vi "TicTacToev3.vi"() -> ()   [LabVIEW 2020]
panel:
  out "Human(GREEN) Win":dbl
  out "Computer(RED)Win":dbl
  in  "Numeric":i32
  out "Who's Tern ?":bool
  in  "LEVEL":i32(slide)=3000 scale=5.0..1.0
  in  "START GAME":bool
  in  "Boolean":bool
  in  "Boolean 3":bool
  in  "Boolean 4":bool
  in  "Boolean 5":bool
  in  "Boolean 6":bool
  in  "Boolean 7":bool
  in  "Boolean 8":bool
  in  "Boolean 9":bool
  in  "Boolean 2":bool
  in  "Turn 2":bool
  out "Turn":string
  out "Human Won":bool
  out "Computer Won":bool
  out "XO array":string[][](array[string])
  out "No one Won":bool
  out "Tie":bool
  in  "STOP GAME":bool
  out "Tank":i32(slide)
  out "Tank 2":i32(slide)
  out "players":dbl format="%#g"
  out "Game Over":bool
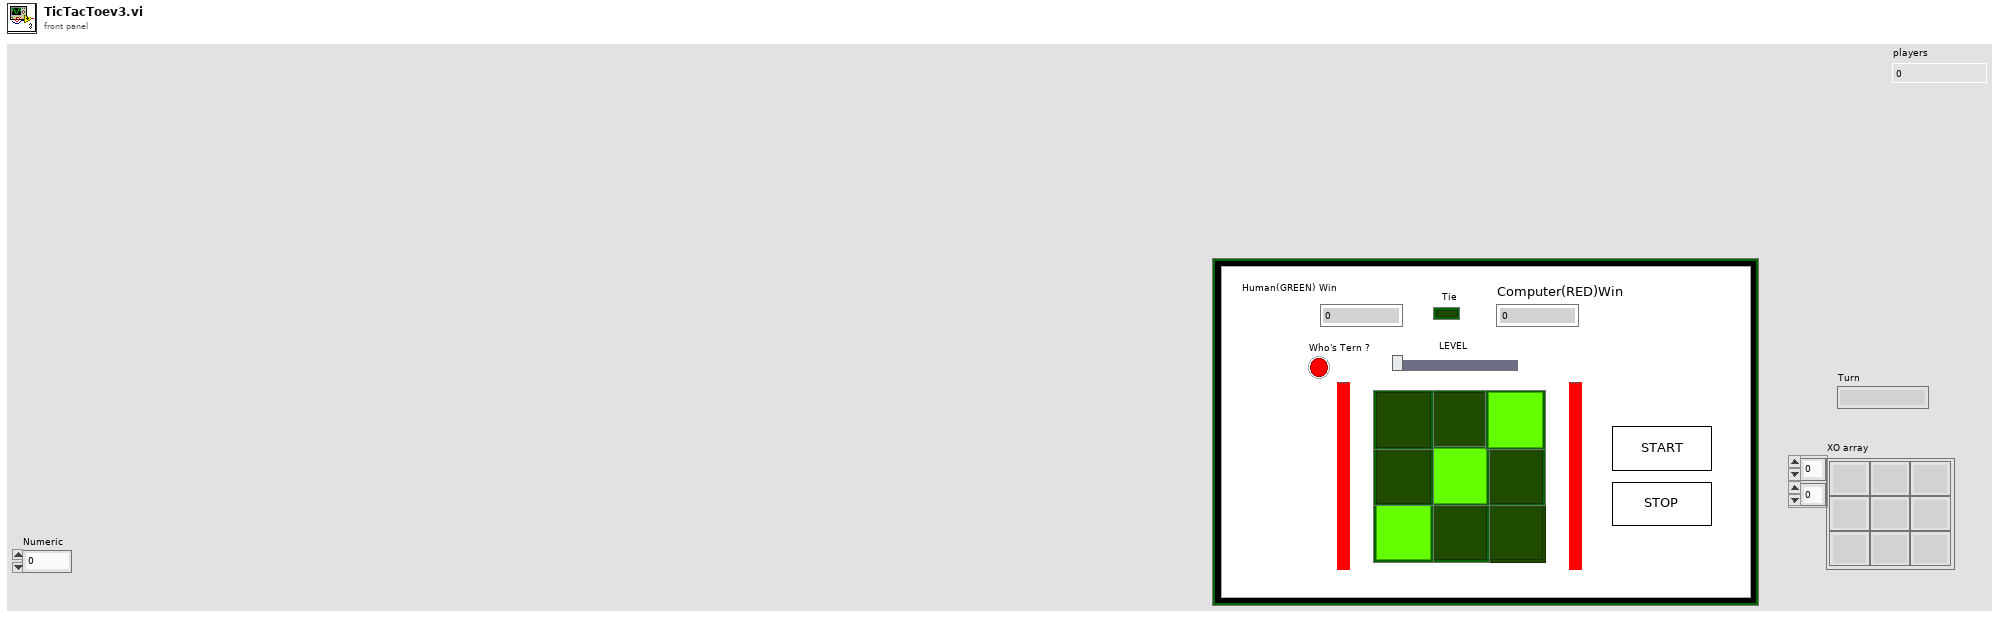
[diagram p1: front panel]
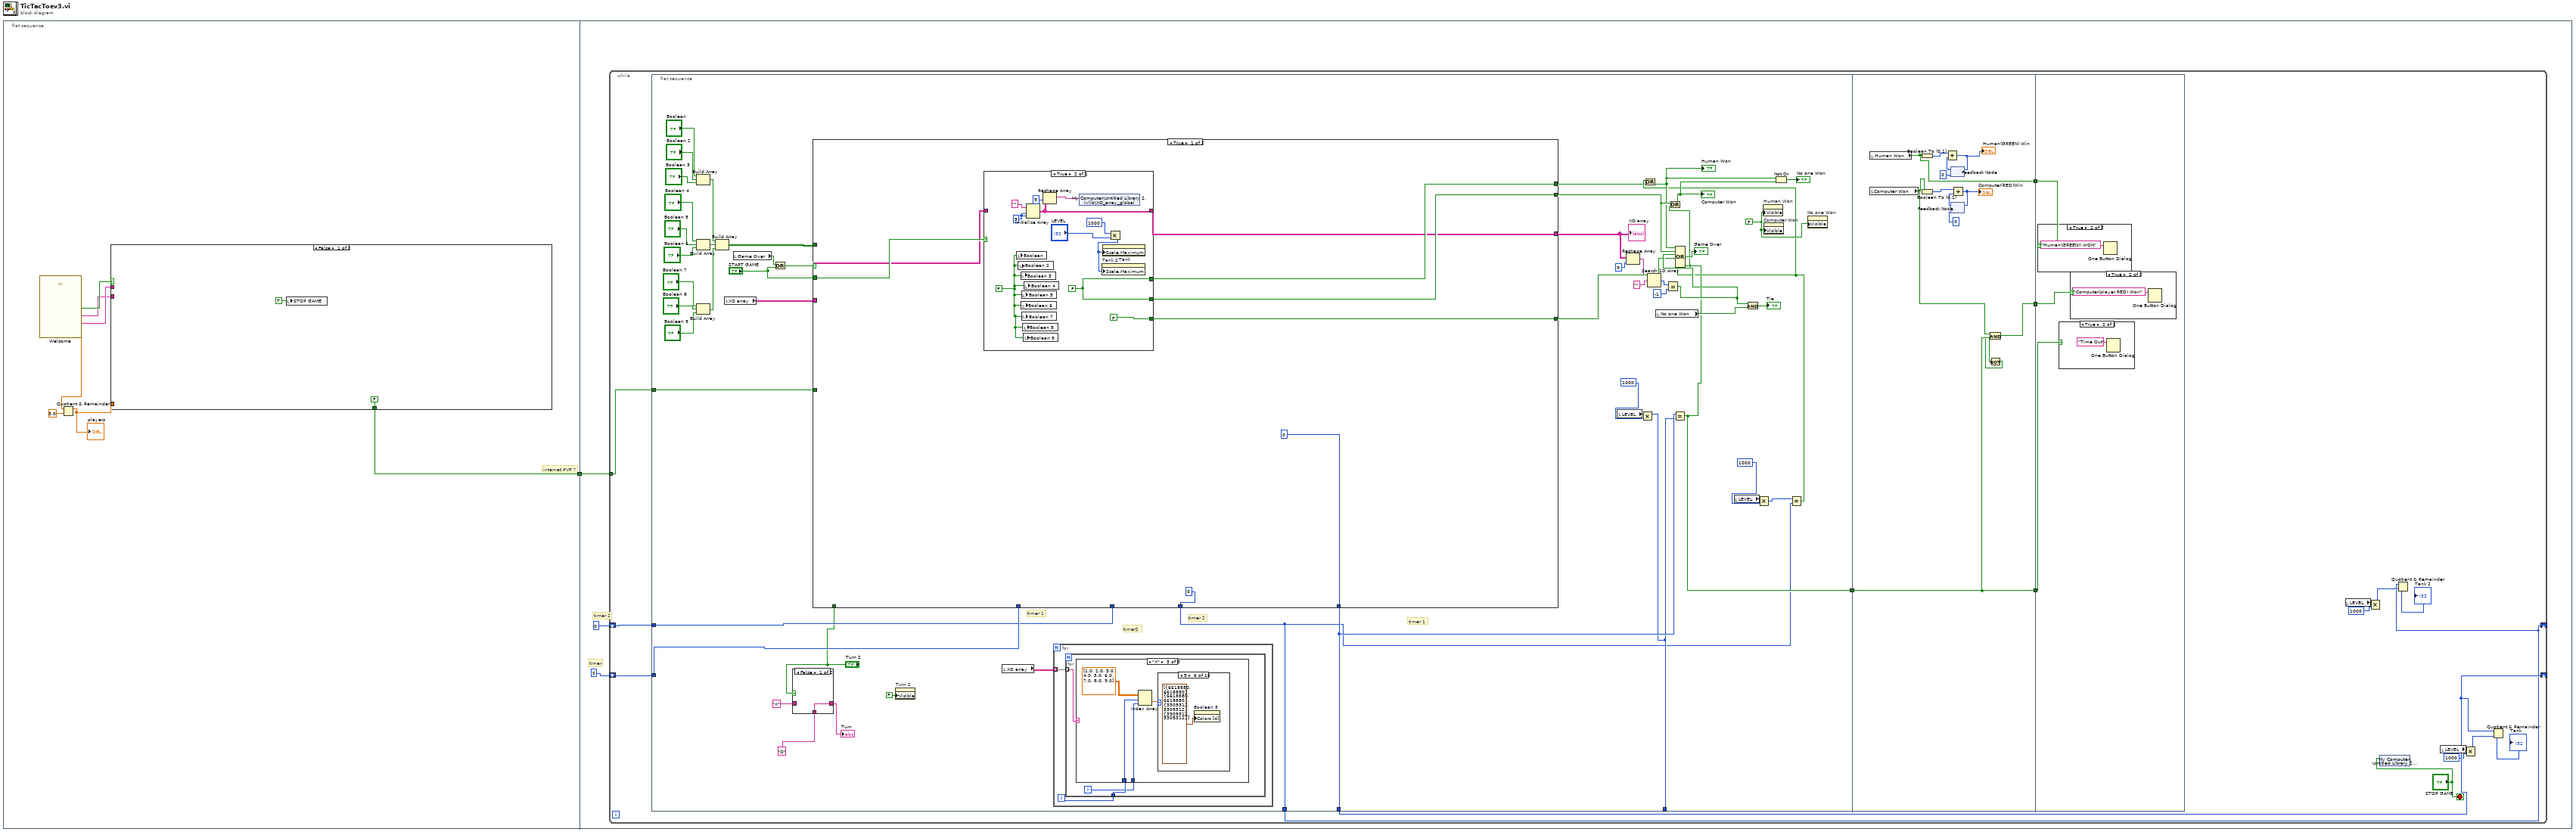
[diagram p0: block diagram]
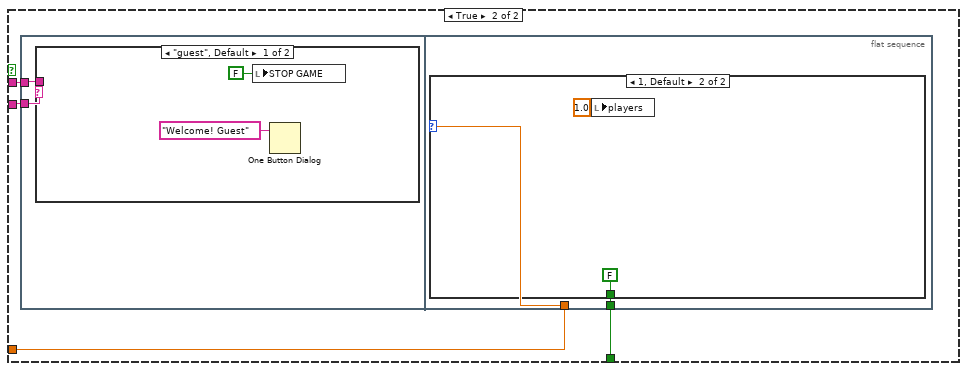
[diagram p2: hidden frame]
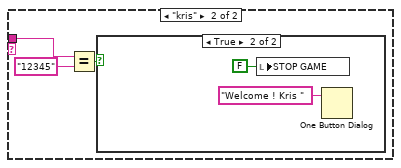
[diagram p3: hidden frame]
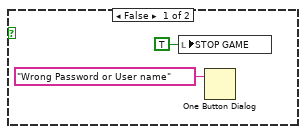
[diagram p4: hidden frame]
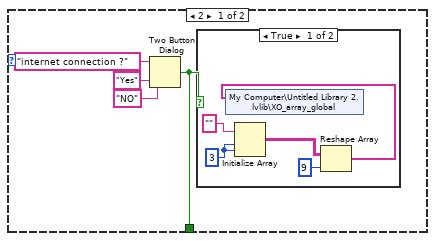
[diagram p5: hidden frame]
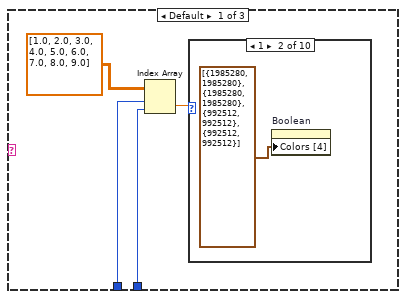
[diagram p7: hidden frame]
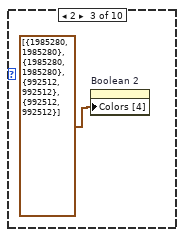
[diagram p9: hidden frame]
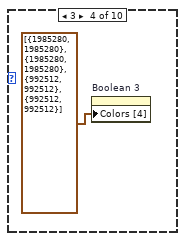
[diagram p10: hidden frame]
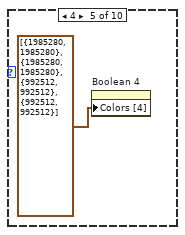
[diagram p11: hidden frame]
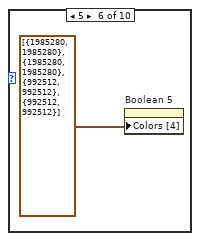
[diagram p12: hidden frame]
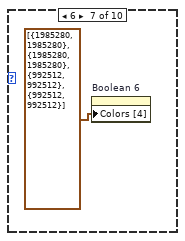
[diagram p13: hidden frame]
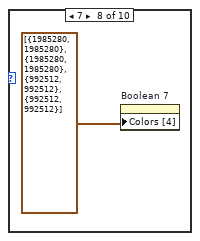
[diagram p14: hidden frame]
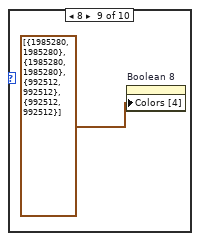
[diagram p15: hidden frame]
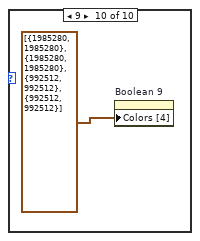
[diagram p16: hidden frame]
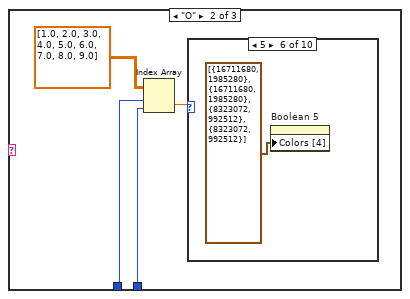
[diagram p17: hidden frame]
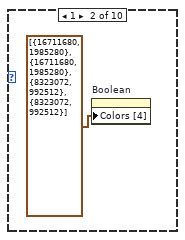
[diagram p19: hidden frame]
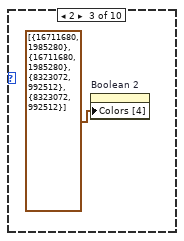
[diagram p20: hidden frame]
diagram:
  n1 = flat-sequence {
    tunnel: [w2] -> w1
    tunnel: w1 -> [w39]
    frame #0 {
      # "internet PVP ?"
      n2 = call "Welcome"() -> ("players(1 or 2 )"=w8:dbl, "password"=w5:string, "name"=w4:string, "OK"=w7:bool)  [unwired: 15 in, 1 out]
      n3 = Quotient & Remainder(x=w8, y=3.0) -> (x-y*floor(x/y)=w3:dbl)  [unwired: 1 out]
      "players" <- w3
      n4 = case shown="False" w7 {
        tunnel: w4 -> [_ w14]
        tunnel: w5 -> [_ w13]
        tunnel: w3 -> [_ w12]
        tunnel: [FALSE ("T button?") w11] -> w2
        frame False {
          n5 = local write "STOP GAME"(TRUE ("STOP GAME")) -> ()
        }
        frame True {
          n6 = flat-sequence {
            tunnel: w14 -> [w16]
            tunnel: w13 -> [w15]
            tunnel: w12 -> [w27]
            tunnel: [w26] -> w11
            frame #0 {
              n7 = case shown="\"guest\", Default" w16 {
                tunnel: w15 -> [_ w21]
                frame "guest", Default {
                  n8 = local write "STOP GAME"(FALSE ("STOP GAME")) -> ()
                  n9 = One Button Dialog(message="Welcome! Guest") -> ()  [unwired: 1 in, 1 out]
                }
                frame "kris" {
                  n10 = Equal?(x=w21, y="12345") -> (x = y?=w19:bool)
                  n11 = case shown="True" w19 {
                    frame False {
                      n12 = local write "STOP GAME"(TRUE ("STOP GAME")) -> ()
                      n13 = One Button Dialog(message="Wrong Password or User name") -> ()  [unwired: 1 in, 1 out]
                    }
                    frame True {
                      n14 = local write "STOP GAME"(FALSE ("STOP GAME")) -> ()
                      n15 = One Button Dialog(message="Welcome ! Kris ") -> ()  [unwired: 1 in, 1 out]
                    }
                  }
                }
              }
            }
            frame #1 {
              n16 = case shown="1, Default" w27 {
                tunnel: [w28 FALSE ("T button?")] -> w26
                frame 2 {
                  n17 = Two Button Dialog(message="internet connection ?", 1:"NO" ("F button name (\"Cancel\")"), 2:"Yes" ("T button name (\"OK\")")) -> (T button?=w28:bool)
                  n18 = case shown="True" w28 {
                    frame True {
                      w36 = 3
                      n19 = Initialize Array("", w36, w36) -> (w33:string[][])
                      n20 = Reshape Array(w33, 9 ("dimension size")) -> (w32:string[])
                      n21 = shared-variable "My Computer\\Untitled Library 2.lvlib\\XO_array_global"(w32) -> ()  [unwired: 1 in, 1 out]
                    }
                    frame False {
                    }
                  }
                }
                frame 1, Default {
                  n22 = local write "players"(1.0 ("players")) -> ()
                }
              }
            }
          }
        }
      }
    }
    frame #1 {
      # "timer 2"
      # "timer"
      n23 = while {
        shift-right: [w55] -> _
        shift-left: 0 -> [w57]
        shift-right: [w44] -> _
        shift-left: 0 -> [w49]
        tunnel: w39 -> [w42]
        stop <- "STOP GAME" stop-if-true
        n24 = flat-sequence {
          tunnel: [w75] -> w55
          tunnel: [w73] -> w53
          tunnel: [w71] -> _
          tunnel: w57 -> [w76]
          tunnel: w49 -> [w69]
          tunnel: [w65] -> w44
          tunnel: w42 -> [w61]
          tunnel: [w323] -> w59
          tunnel: [w326] -> w58
          tunnel: [w325] -> w54
          tunnel: w53 -> [w325]
          tunnel: w59 -> [w337]
          tunnel: w58 -> [w336]
          tunnel: w54 -> [w335]
          frame #0 {
            w78 = FALSE ("Visible")
            # "timer 1"
            # "timer 2"
            # "timer 1"
            # "timer2"
            n25 = Build Array("Boolean", "Boolean 2", "Boolean 3") -> (w110:bool[])
            n26 = Build Array("Boolean 4", "Boolean 5", "Boolean 6") -> (w111:bool[])
            n27 = Build Array("Boolean 7", "Boolean 8", "Boolean 9") -> (w112:bool[])
            n28 = Build Array(w110, w111, w112) -> (w102:bool[][])
            n29 = local read "XO array"() -> (w101:string[][])
            n30 = local read "Game Over"() -> (w94:bool)
            n31 = Or(x=w94, y="START GAME") -> (x .or. y?=w93:bool)
            n32 = case shown="False" "Turn 2" {
              tunnel: "X" -> [_ w158]
              tunnel: [w157 w158] -> w99
              tunnel: "O" ("x") -> [w157 _]
              frame False {
              }
              frame True {
              }
            }
            "Turn" <- w99
            n33 = case shown="True" w93 {
              tunnel: w102 -> [_ w202]
              tunnel: w101 -> [w165 w181]
              tunnel: "Turn 2" -> [_ w201]
              tunnel: "START GAME" -> [w166 _]
              tunnel: [w164 w194] -> w80
              tunnel: [w163 w193] -> w79
              tunnel: [w162 w192] -> w83
              tunnel: [w161 FALSE] -> w77
              tunnel: w76 -> [_ w190]
              tunnel: [0 w189] -> w75
              tunnel: w69 -> [_ w188]
              tunnel: [0 w187] -> w65
              tunnel: w61 -> [_ w183]
              frame True {
                n34 = case shown="True" w166 {
                  tunnel: [w169 w172] -> w162
                  tunnel: [w168 w179] -> w163
                  tunnel: [w168 w179] -> w164
                  tunnel: w165 -> [w169 _]
                  tunnel: [TRUE FALSE] -> w161
                  frame False {
                    w168 = FALSE
                  }
                  frame True {
                    w177 = FALSE
                    w179 = FALSE
                    w178 = 3
                    n35 = local write "Boolean"(w177) -> ()
                    n36 = local write "Boolean 2"(w177) -> ()
                    n37 = local write "Boolean 3"(w177) -> ()
                    n38 = local write "Boolean 6"(w177) -> ()
                    n39 = local write "Boolean 5"(w177) -> ()
                    n40 = local write "Boolean 7"(w177) -> ()
                    n41 = local write "Boolean 8"(w177) -> ()
                    n42 = local write "Boolean 9"(w177) -> ()
                    n43 = local write "Boolean 4"(w177) -> ()
                    n44 = Initialize Array("", w178, w178) -> (w172:string[][])
                    n45 = Reshape Array(w172, 9 ("dimension size")) -> (w171:string[])
                    n46 = shared-variable "My Computer\\Untitled Library 2.lvlib\\XO_array_global"(w171) -> ()  [unwired: 1 in, 1 out]
                    n47 = Multiply(x=1000, y="LEVEL") -> (x*y=w173:i32)
                    n48 = property on="Tank 2" class="Slide (strict)"("Scale.Maximum"=w173) -> ()  [unwired: 2 in, 2 out]
                    n49 = property on="Tank" class="Slide (strict)"("Scale.Maximum"=w173) -> ()  [unwired: 2 in, 2 out]
                  }
                }
              }
              frame False {
                n50 = local read "Turn"() -> (w182:string)
                n51 = shared-variable "My Computer\\Untitled Library 2.lvlib\\Turn_string"(w182) -> ()  [unwired: 1 in, 1 out]
                n52 = Equal?(x=w182, y="O") -> (x = y?=w185:bool)
                n53 = case shown="False" w185 {
                  frame False {
                    n54 = property on="Who's Tern ?" class="Bool (strict)"("Colors [4]"=cluster{u32, u32}[] [{6618880, 6618880}]) -> ()  [unwired: 2 in, 2 out]
                  }
                  frame True {
                    n55 = property on="Who's Tern ?" class="Bool (strict)"("Colors [4]"=cluster{u32, u32}[] [{16711680, 16711680}]) -> ()  [unwired: 2 in, 2 out]
                  }
                }
                n56 = case shown="False" w201 {
                  selector: w201 -> [w209 _]
                  tunnel: w202 -> [w216 w292]
                  tunnel: w181 -> [w218 w291]
                  tunnel: [w219 w284] -> w192
                  tunnel: w182 -> [w215 w290]
                  tunnel: w190 -> [w211 w288]
                  tunnel: [w214 w287] -> w189
                  tunnel: w188 -> [w213 _]
                  tunnel: [w212 0] -> w187
                  tunnel: w183 -> [w210 _]
                  frame False {
                    n57 = local read "players"() -> (w217:dbl)
                    n58 = case shown="2" w217 {
                      tunnel: [w225 w281] -> w219
                      tunnel: w218 -> [w228 w280]
                      tunnel: w216 -> [w226 _]
                      tunnel: w215 -> [w227 _]
                      tunnel: w213 -> [w224 _]
                      tunnel: [0 0] -> w214
                      tunnel: [w223 0] -> w212
                      tunnel: w211 -> [_ _]
                      tunnel: w210 -> [w221 _]
                      tunnel: w209 -> [w220 _]
                      frame 2 {
                        # "connect to timer2"
                        n59 = case shown="True" w221 {
                          tunnel: w228 -> [_ w245]
                          tunnel: w227 -> [_ w244]
                          tunnel: w226 -> [_ w243]
                          tunnel: [w231 w242] -> w225
                          tunnel: w224 -> [_ w241]
                          tunnel: ["Numeric" w240] -> w223
                          tunnel: w220 -> [w229 _]
                          frame True {
                            n60 = flat-sequence {
                              tunnel: w229 -> [w232]
                              tunnel: [w238] -> w231
                              frame #0 {
                                n61 = shared-variable "My Computer\\Untitled Library 2.lvlib\\Internet_PVP"(TRUE ("Internet_PVP")) -> ()  [unwired: 1 in, 1 out]
                                n62 = shared-variable "My Computer\\Untitled Library 2.lvlib\\Turn"(w232) -> ()  [unwired: 1 in, 1 out]
                                n63 = shared-variable "My Computer\\Untitled Library 2.lvlib\\timer_2"() -> (w233:i32)  [unwired: 1 in, 1 out]
                                n64 = local write "Numeric"(w233) -> ()
                              }
                              frame #1 {
                                n65 = shared-variable "My Computer\\Untitled Library 2.lvlib\\XO_array_global"() -> (w239:string[])  [unwired: 1 in, 1 out]
                                n66 = shared-variable "My Computer\\Untitled Library 2.lvlib\\Client_end"() -> (w235:bool)  [unwired: 1 in, 1 out]
                                n67 = local write "Turn 2"(w235) -> ()
                                n68 = Reshape Array(w239, 3 ("dimension size"), 3 ("dimension size")) -> (w238:string[][])
                              }
                            }
                          }
                          frame False {
                            w246 = 3
                            n69 = for {
                              N: w246 -> [_]
                              tunnel: w246 -> [w253]
                              tunnel: w243 -> [w252] mode=indexing
                              tunnel: w245 -> [w251] mode=indexing
                              tunnel: [w250] -> w242 mode=indexing
                              tunnel: w244 -> [w249]
                              tunnel: w241 -> [w248]
                              tunnel: [w247] -> w240
                              n70 = for {
                                N: w253 -> [_]
                                tunnel: w252 -> [w263] mode=indexing
                                tunnel: w251 -> [w260] mode=indexing
                                tunnel: w249 -> [w258]
                                tunnel: [w259] -> w250 mode=indexing
                                tunnel: w248 -> [w255]
                                tunnel: [w254] -> w247
                                n71 = Not Equal?(x=w260, y="X") -> (x != y?=w264:bool)
                                n72 = Not Equal?(x="O", y=w260) -> (x != y?=w265:bool)
                                n73 = And(x=w265, y=w264) -> (x .and. y?=w262:bool)
                                n74 = local read "Turn 2"() -> (w257:bool)
                                n75 = And(x=w263, y=w262) -> (x .and. y?=w261:bool)
                                n76 = case shown="True" w261 {
                                tunnel: w260 -> [w271 _]
                                tunnel: [w271 w273] -> w259
                                tunnel: w258 -> [_ w273]
                                tunnel: [w270 w274] -> w256
                                tunnel: w257 -> [w270 w275]
                                tunnel: w255 -> [w269 _]
                                tunnel: [w268 0] -> w254
                                frame False {
                                n77 = Increment(x=w269) -> (x+1=w268:i32)
                                }
                                frame True {
                                n78 = Not(x=w275) -> (.not. x?=w274:bool)
                                }
                                }
                                n79 = local write "Turn 2"(w256) -> ()
                              }
                            }
                          }
                        }
                      }
                      frame 1, Default {
                        n80 = local read "Turn 2"() -> (w279:bool)
                        n81 = call "AI algorithm(SubVI).vi"("Turn"=w279, "XO array"=w280) -> ("Turn 2"=w278:bool, "XO array 2"=w281:string[][])
                        n82 = local write "Turn 2"(w278) -> ()
                      }
                    }
                  }
                  frame True {
                    w289 = 3
                    n83 = for {
                      N: w289 -> [_]
                      tunnel: w289 -> [w299]
                      tunnel: w292 -> [w298] mode=indexing
                      tunnel: w291 -> [w297] mode=indexing
                      tunnel: [w296] -> w284 mode=indexing
                      tunnel: w290 -> [w295]
                      tunnel: w288 -> [w294]
                      tunnel: [w293] -> w287
                      n84 = for {
                        N: w299 -> [_]
                        tunnel: w298 -> [w309] mode=indexing
                        tunnel: w297 -> [w307] mode=indexing
                        tunnel: w295 -> [w305]
                        tunnel: [w306] -> w296 mode=indexing
                        tunnel: w294 -> [w301]
                        tunnel: [w300] -> w293
                        n85 = Not Equal?(x=w307, y="X") -> (x != y?=w310:bool)
                        n86 = Not Equal?(x="O", y=w307) -> (x != y?=w311:bool)
                        n87 = And(x=w311, y=w310) -> (x .and. y?=w308:bool)
                        n88 = local read "Turn 2"() -> (w303:bool)
                        n89 = And(x=w309, y=w308) -> (x .and. y?=w302:bool)
                        n90 = case shown="False" w302 {
                          tunnel: w307 -> [w317 _]
                          tunnel: [w317 w319] -> w306
                          tunnel: w305 -> [_ w319]
                          tunnel: [w316 w320] -> w304
                          tunnel: w303 -> [w316 w321]
                          tunnel: w301 -> [w315 _]
                          tunnel: [w314 0] -> w300
                          frame False {
                            n91 = Increment(x=w315) -> (x+1=w314:i32)
                          }
                          frame True {
                            n92 = Not(x=w321) -> (.not. x?=w320:bool)
                          }
                        }
                        n93 = local write "Turn 2"(w304) -> ()
                      }
                    }
                    n94 = shared-variable "My Computer\\Untitled Library 2.lvlib\\timer_2"(0 ("timer_2")) -> ()  [unwired: 1 in, 1 out]
                    n95 = Reshape Array(w284, 9 ("dimension size")) -> (w282:string[])
                    n96 = shared-variable "My Computer\\Untitled Library 2.lvlib\\XO_array_global"(w282) -> ()  [unwired: 1 in, 1 out]
                  }
                }
                n97 = call "CheckWinDiag(SubVI).vi"("Array"=w192) -> ("x .or. y?"=w199:bool)  [unwired: 10 in]
                n98 = Transpose 2D Array(2D array=w192) -> (transposed array=w200:string[][])
                n99 = call "CheckWinRow(SubVI).vi"("Array"=w192) -> ("x .or. y? 2"=w198:bool)  [unwired: 10 in]
                n100 = call "CheckWinRow(SubVI).vi"("Array"=w200) -> ("x .or. y? 2"=w197:bool)  [unwired: 10 in]
                n101 = local read "Turn"() -> (w195:string)
                n102 = Compound Arithmetic op=OR(w199, w198, w197) -> (w196:bool)
                n103 = case shown="\"O\", Default" w195 {
                  tunnel: w196 -> [w206 w207]
                  tunnel: [w206 FALSE] -> w194
                  tunnel: [FALSE w207] -> w193
                  frame "O", Default {
                  }
                  frame "X" {
                  }
                }
                "Who's Tern ?" <- TRUE ("Boolean 10")
              }
            }
            "XO array" <- w83
            n104 = property on="Turn 2" class="Bool (strict)"("Visible"=FALSE) -> ()  [unwired: 2 in, 2 out]
            n105 = local read "XO array"() -> (w82:string[][])
            n106 = for {
              tunnel: w82 -> [w113] mode=indexing
              i -> [w114]
              n107 = for {
                tunnel: w114 -> [w117]
                tunnel: w113 -> [w115] mode=indexing
                i -> [w116]
                n108 = case shown="\"X\"" w115 {
                  tunnel: w117 -> [w121 w132 w145]
                  tunnel: w116 -> [w120 w131 w146]
                  frame Default {
                    n109 = Index Array(array=dbl[][] [[1.0, 2.0, 3.0], [4.0, 5.0, 6.0], [7.0, 8.0, 9.0]] ("Array"), index (row)=w121, index (col)=w120) -> (element=w118:dbl)
                    n110 = case shown="1" w118 {
                      frame 0, Default {
                      }
                      frame 1 {
                        n111 = property on="Boolean" class="Bool (strict)"("Colors [4]"=cluster{u32, u32}[] [{1985280, 1985280}, {1985280, 1985280}, {992512, 992512}, {992512, 992512}]) -> ()  [unwired: 2 in, 2 out]
                      }
                      frame 2 {
                        n112 = property on="Boolean 2" class="Bool (strict)"("Colors [4]"=cluster{u32, u32}[] [{1985280, 1985280}, {1985280, 1985280}, {992512, 992512}, {992512, 992512}]) -> ()  [unwired: 2 in, 2 out]
                      }
                      frame 3 {
                        n113 = property on="Boolean 3" class="Bool (strict)"("Colors [4]"=cluster{u32, u32}[] [{1985280, 1985280}, {1985280, 1985280}, {992512, 992512}, {992512, 992512}]) -> ()  [unwired: 2 in, 2 out]
                      }
                      frame 4 {
                        n114 = property on="Boolean 4" class="Bool (strict)"("Colors [4]"=cluster{u32, u32}[] [{1985280, 1985280}, {1985280, 1985280}, {992512, 992512}, {992512, 992512}]) -> ()  [unwired: 2 in, 2 out]
                      }
                      frame 5 {
                        n115 = property on="Boolean 5" class="Bool (strict)"("Colors [4]"=cluster{u32, u32}[] [{1985280, 1985280}, {1985280, 1985280}, {992512, 992512}, {992512, 992512}]) -> ()  [unwired: 2 in, 2 out]
                      }
                      frame 6 {
                        n116 = property on="Boolean 6" class="Bool (strict)"("Colors [4]"=cluster{u32, u32}[] [{1985280, 1985280}, {1985280, 1985280}, {992512, 992512}, {992512, 992512}]) -> ()  [unwired: 2 in, 2 out]
                      }
                      frame 7 {
                        n117 = property on="Boolean 7" class="Bool (strict)"("Colors [4]"=cluster{u32, u32}[] [{1985280, 1985280}, {1985280, 1985280}, {992512, 992512}, {992512, 992512}]) -> ()  [unwired: 2 in, 2 out]
                      }
                      frame 8 {
                        n118 = property on="Boolean 8" class="Bool (strict)"("Colors [4]"=cluster{u32, u32}[] [{1985280, 1985280}, {1985280, 1985280}, {992512, 992512}, {992512, 992512}]) -> ()  [unwired: 2 in, 2 out]
                      }
                      frame 9 {
                        n119 = property on="Boolean 9" class="Bool (strict)"("Colors [4]"=cluster{u32, u32}[] [{1985280, 1985280}, {1985280, 1985280}, {992512, 992512}, {992512, 992512}]) -> ()  [unwired: 2 in, 2 out]
                      }
                    }
                  }
                  frame "O" {
                    n120 = Index Array(array=dbl[][] [[1.0, 2.0, 3.0], [4.0, 5.0, 6.0], [7.0, 8.0, 9.0]] ("Array"), index (row)=w132, index (col)=w131) -> (element=w133:dbl)
                    n121 = case shown="5" w133 {
                      frame 0, Default {
                      }
                      frame 1 {
                        n122 = property on="Boolean" class="Bool (strict)"("Colors [4]"=cluster{u32, u32}[] [{16711680, 1985280}, {16711680, 1985280}, {8323072, 992512}, {8323072, 992512}]) -> ()  [unwired: 2 in, 2 out]
                      }
                      frame 2 {
                        n123 = property on="Boolean 2" class="Bool (strict)"("Colors [4]"=cluster{u32, u32}[] [{16711680, 1985280}, {16711680, 1985280}, {8323072, 992512}, {8323072, 992512}]) -> ()  [unwired: 2 in, 2 out]
                      }
                      frame 3 {
                        n124 = property on="Boolean 3" class="Bool (strict)"("Colors [4]"=cluster{u32, u32}[] [{16711680, 1985280}, {16711680, 1985280}, {8323072, 992512}, {8323072, 992512}]) -> ()  [unwired: 2 in, 2 out]
                      }
                      frame 4 {
                        n125 = property on="Boolean 4" class="Bool (strict)"("Colors [4]"=cluster{u32, u32}[] [{16711680, 1985280}, {16711680, 1985280}, {8323072, 992512}, {8323072, 992512}]) -> ()  [unwired: 2 in, 2 out]
                      }
                      frame 5 {
                        n126 = property on="Boolean 5" class="Bool (strict)"("Colors [4]"=cluster{u32, u32}[] [{16711680, 1985280}, {16711680, 1985280}, {8323072, 992512}, {8323072, 992512}]) -> ()  [unwired: 2 in, 2 out]
                      }
                      frame 6 {
                        n127 = property on="Boolean 6" class="Bool (strict)"("Colors [4]"=cluster{u32, u32}[] [{16711680, 1985280}, {16711680, 1985280}, {8323072, 992512}, {8323072, 992512}]) -> ()  [unwired: 2 in, 2 out]
                      }
                      frame 7 {
                        n128 = property on="Boolean 7" class="Bool (strict)"("Colors [4]"=cluster{u32, u32}[] [{16711680, 1985280}, {16711680, 1985280}, {8323072, 992512}, {8323072, 992512}]) -> ()  [unwired: 2 in, 2 out]
                      }
                      frame 8 {
                        n129 = property on="Boolean 8" class="Bool (strict)"("Colors [4]"=cluster{u32, u32}[] [{16711680, 1985280}, {16711680, 1985280}, {8323072, 992512}, {8323072, 992512}]) -> ()  [unwired: 2 in, 2 out]
                      }
                      frame 9 {
                        n130 = property on="Boolean 9" class="Bool (strict)"("Colors [4]"=cluster{u32, u32}[] [{16711680, 1985280}, {16711680, 1985280}, {8323072, 992512}, {8323072, 992512}]) -> ()  [unwired: 2 in, 2 out]
                      }
                    }
                  }
                  frame "X" {
                    n131 = Index Array(array=dbl[][] [[1.0, 2.0, 3.0], [4.0, 5.0, 6.0], [7.0, 8.0, 9.0]] ("Array"), index (row)=w145, index (col)=w146) -> (element=w147:dbl)
                    n132 = case shown="5" w147 {
                      frame 0, Default {
                      }
                      frame 1 {
                        n133 = property on="Boolean" class="Bool (strict)"("Colors [4]"=cluster{u32, u32}[] [{6618880, 6618880}, {6618880, 6618880}, {3309312, 3309312}, {3309312, 3309312}]) -> ()  [unwired: 2 in, 2 out]
                      }
                      frame 2 {
                        n134 = property on="Boolean 2" class="Bool (strict)"("Colors [4]"=cluster{u32, u32}[] [{6618880, 6618880}, {6618880, 6618880}, {3309312, 3309312}, {3309312, 3309312}]) -> ()  [unwired: 2 in, 2 out]
                      }
                      frame 3 {
                        n135 = property on="Boolean 3" class="Bool (strict)"("Colors [4]"=cluster{u32, u32}[] [{6618880, 6618880}, {6618880, 6618880}, {3309312, 3309312}, {3309312, 3309312}]) -> ()  [unwired: 2 in, 2 out]
                      }
                      frame 4 {
                        n136 = property on="Boolean 4" class="Bool (strict)"("Colors [4]"=cluster{u32, u32}[] [{6618880, 6618880}, {6618880, 6618880}, {3309312, 3309312}, {3309312, 3309312}]) -> ()  [unwired: 2 in, 2 out]
                      }
                      frame 5 {
                        n137 = property on="Boolean 5" class="Bool (strict)"("Colors [4]"=cluster{u32, u32}[] [{6618880, 6618880}, {6618880, 6618880}, {3309312, 3309312}, {3309312, 3309312}]) -> ()  [unwired: 2 in, 2 out]
                      }
                      frame 6 {
                        n138 = property on="Boolean 6" class="Bool (strict)"("Colors [4]"=cluster{u32, u32}[] [{6618880, 6618880}, {6618880, 6618880}, {3309312, 3309312}, {3309312, 3309312}]) -> ()  [unwired: 2 in, 2 out]
                      }
                      frame 7 {
                        n139 = property on="Boolean 7" class="Bool (strict)"("Colors [4]"=cluster{u32, u32}[] [{6618880, 6618880}, {6618880, 6618880}, {3309312, 3309312}, {3309312, 3309312}]) -> ()  [unwired: 2 in, 2 out]
                      }
                      frame 8 {
                        n140 = property on="Boolean 8" class="Bool (strict)"("Colors [4]"=cluster{u32, u32}[] [{6618880, 6618880}, {6618880, 6618880}, {3309312, 3309312}, {3309312, 3309312}]) -> ()  [unwired: 2 in, 2 out]
                      }
                      frame 9 {
                        n141 = property on="Boolean 9" class="Bool (strict)"("Colors [4]"=cluster{u32, u32}[] [{6618880, 6618880}, {6618880, 6618880}, {3309312, 3309312}, {3309312, 3309312}]) -> ()  [unwired: 2 in, 2 out]
                      }
                    }
                  }
                }
              }
            }
            n142 = local read "LEVEL"() -> (w72:i32)
            n143 = Reshape Array(w83, 9 ("dimension size")) -> (w62:string[])
            n144 = Multiply(x=w72, y=1000) -> (x*y=w71:i32)
            n145 = Search 1D Array(1D array=w62, element="") -> (index of element=w87:i32)  [unwired: 1 in]
            n146 = local read "No one Won"() -> (w90:bool)
            n147 = Equal?(x=w87, y=-1) -> (x = y?=w84:bool)
            n148 = Equal?(x=w75, y=w71) -> (x = y?=w73:bool)
            n149 = Or(x=w80, y=w73) -> (x .or. y?=w74:bool)
            "Computer Won" <- w74
            n150 = local read "LEVEL"() -> (w67:i32)
            n151 = And(x=w84, y=w90) -> (x .and. y?=→"Tie":bool)
            n152 = Multiply(x=w67, y=1000) -> (x*y=w66:i32)
            n153 = property on="Human Won" class="Bool (strict)"("Visible"=w78) -> ()  [unwired: 2 in, 2 out]
            n154 = property on="Computer Won" class="Bool (strict)"("Visible"=w78) -> ()  [unwired: 2 in, 2 out]
            n155 = Equal?(x=w66, y=w65) -> (x = y?=w63:bool)
            n156 = Or(x=w63, y=w79) -> (x .or. y?=w64:bool)
            "Human Won" <- w64
            n157 = Compound Arithmetic op=OR(w64, w80, w84, w77, w73, w63) -> (→"Game Over":bool)
            n158 = Not Or(1:w74, 2:w64) -> (0:→"No one Won":bool)
            n159 = property on="No one Won" class="Bool (strict)"("Visible"=w78) -> ()  [unwired: 2 in, 2 out]
          }
          frame #1 {
            n160 = local read "Computer Won"() -> (w324:bool)
            n161 = local read "Human Won"() -> (w326:bool)
            n162 = Boolean To (0,1)(Boolean=w326) -> (0, 1=w329:i16)
            n163 = Boolean To (0,1)(Boolean=w324) -> (0, 1=w327:i16)
            n164 = feedback #1(i16 0) -> (w330:i16)
            n165 = Add(x=w329, y=w330) -> (x+y=w332:i16)
            "Human(GREEN) Win" <- w332
            n166 = feedback-in #1(w332) -> ()
            n167 = feedback #2(i16 0) -> (w328:i16)
            n168 = Add(x=w327, y=w328) -> (x+y=w331:i16)
            "Computer(RED)Win" <- w331
            n169 = feedback-in #2(w331) -> ()
            n170 = Not(x=w325) -> (.not. x?=w322:bool)
            n171 = And(x=w324, y=w322) -> (x .and. y?=w323:bool)
          }
          frame #2 {
            n172 = case shown="True" w336 {
              frame False {
              }
              frame True {
                n173 = One Button Dialog(message="Human(GREEN)) WON") -> ()  [unwired: 1 in, 1 out]
              }
            }
            n174 = case shown="True" w335 {
              frame False {
              }
              frame True {
                n175 = One Button Dialog(message="Time Out") -> ()  [unwired: 1 in, 1 out]
              }
            }
            n176 = case shown="True" w337 {
              frame False {
              }
              frame True {
                n177 = One Button Dialog(message="Computer(player RED) Won") -> ()  [unwired: 1 in, 1 out]
              }
            }
          }
        }
        n178 = local read "LEVEL"() -> (w46:i32)
        n179 = Multiply(x=w46, y=1000) -> (x*y=w47:i32)
        n180 = shared-variable "My Computer\\Untitled Library 2.lvlib\\stop"("STOP GAME") -> ()  [unwired: 1 in, 1 out]
        n181 = Quotient & Remainder(x=w44, y=w47) -> (x-y*floor(x/y)=→"Tank 2":i32)  [unwired: 1 out]
        n182 = local read "LEVEL"() -> (w52:i32)
        n183 = Multiply(x=w52, y=1000) -> (x*y=w51:i32)
        n184 = Quotient & Remainder(x=w55, y=w51) -> (x-y*floor(x/y)=→"Tank":i32)  [unwired: 1 out]
      }
    }
  }
